vi "EMV Offset From Target.vi"(8 "error in (no error)":errorcluster, 10 "User Setpoint Temperature":u16=125, 11 "Current T6 Temperatures":dbl[](array[numeric])) -> (0 "error out":errorcluster, 1 "Absolute T6 Offset From Target 3":dbl, 2 "Absolute T6 Offset From Target 2":dbl, 3 "Absolute T6 Offset From Target 1":dbl)   [LabVIEW 2020]
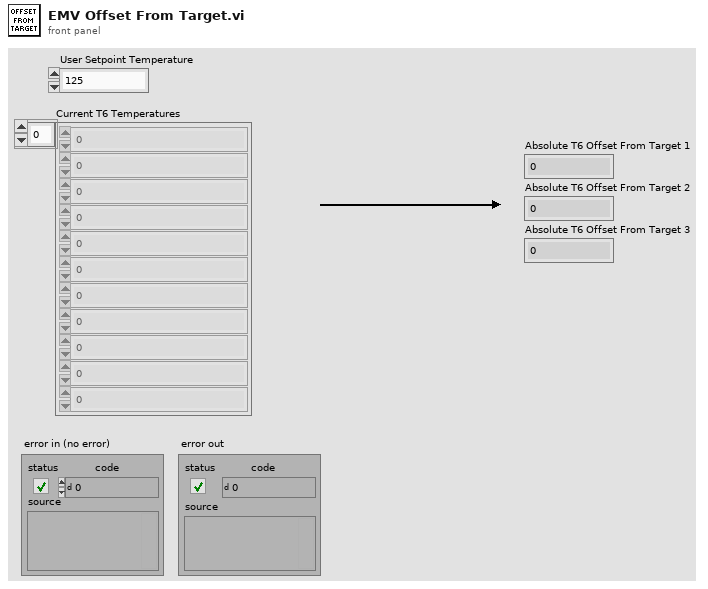
[diagram p1: front panel]
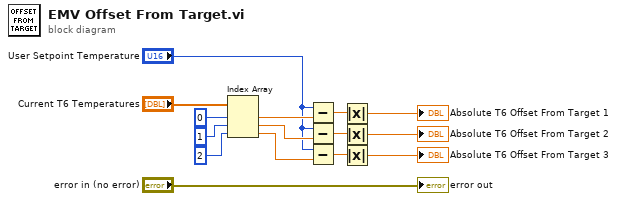
[diagram p0: block diagram]
diagram:
  n1 = Index Array(array="Current T6 Temperatures", index #1=0 ("index"), index #2=1 ("index"), index #3=2 ("index")) -> (element #1=w14:dbl, element #2=w7:dbl, element #3=w6:dbl)
  n2 = Subtract(x="User Setpoint Temperature", y=w14) -> (x-y=w11:dbl)
  n3 = Subtract(x="User Setpoint Temperature", y=w7) -> (x-y=w4:dbl)
  n4 = Subtract(x="User Setpoint Temperature", y=w6) -> (x-y=w3:dbl)
  n5 = Absolute Value(x=w11) -> (abs(x)=→"Absolute T6 Offset From Target 1":dbl)
  n6 = Absolute Value(x=w4) -> (abs(x)=→"Absolute T6 Offset From Target 2":dbl)
  n7 = Absolute Value(x=w3) -> (abs(x)=→"Absolute T6 Offset From Target 3":dbl)
  "error out" <- "error in (no error)"
